vi "All SubFunctions Mod.vi"(4 "מק\"ט המכלל":string, 5 "מספר סידורי":string, 7 "מפעיל":string="ANS", 8 "error":errorcluster, 10 "שם הממסר":string="0410-24534 15A ממסר", 11 "Path for Log":path) -> (0 "error IO":errorcluster)   [LabVIEW 2015]
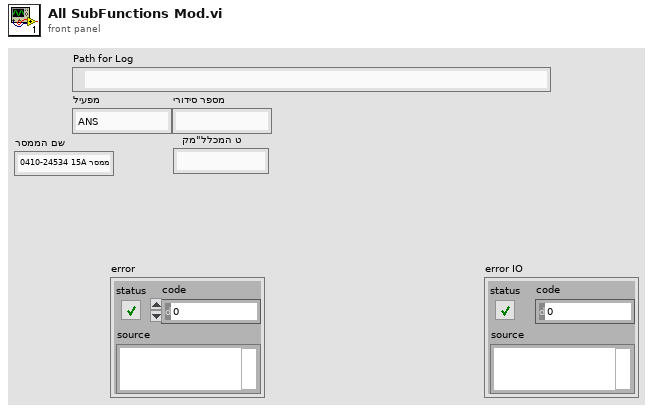
[diagram p1: front panel]
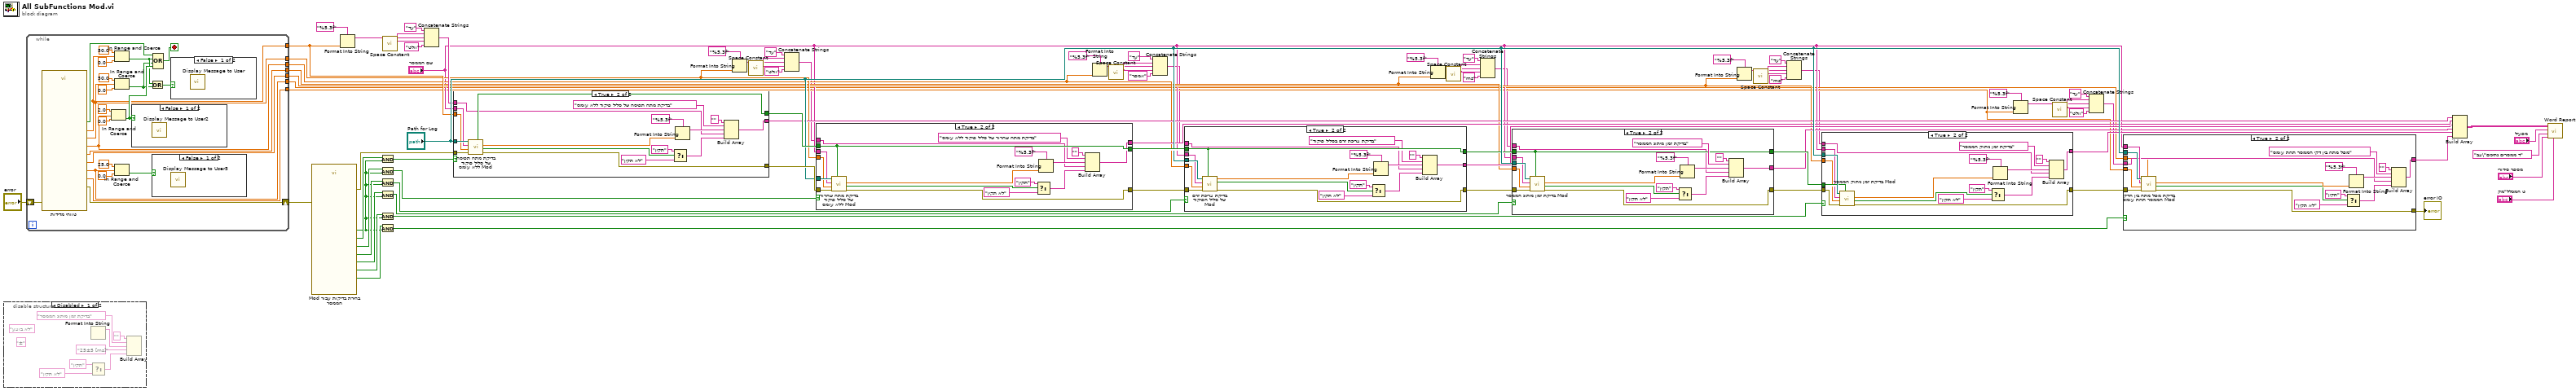
[diagram p0: block diagram]
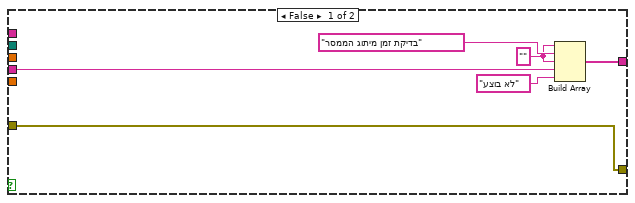
[diagram p6: hidden frame]
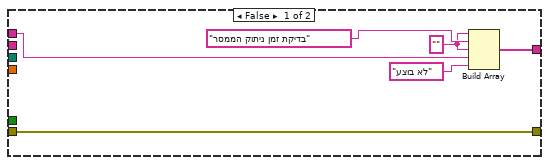
[diagram p7: hidden frame]
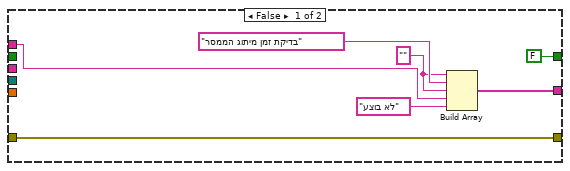
[diagram p8: hidden frame]
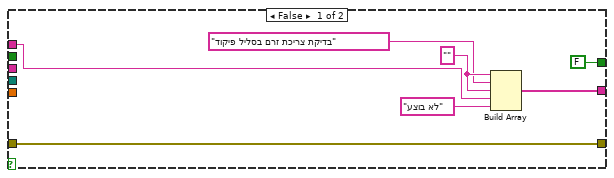
[diagram p9: hidden frame]
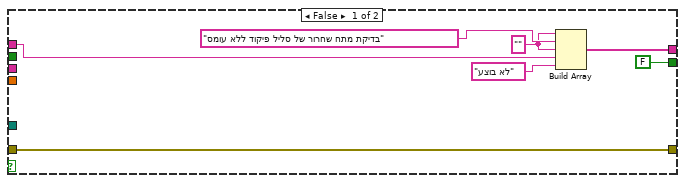
[diagram p10: hidden frame]
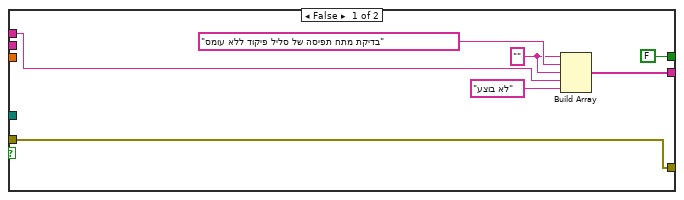
[diagram p11: hidden frame]
diagram:
  n1 = disable-structure shown="Disabled" {
    frame Disabled {
      (unwired) "±"
      (unwired) "לא בוצע"
      n2 = Format Into String() -> (resulting string=w87:string)  [unwired: 4 in, 1 out]
      n3 = Select(t="תקין", f="לא תקין") -> (s? t:f=w89:string)  [unwired: 1 in]
      n4 = Build Array("" ("element"), "בדיקת זמן מיתוג הממסר" ("element"), w87, "25±5 [ms]" ("element"), w89) -> ()  [unwired: 1 out]
    }
    frame Enabled {
    }
  }
  n5 = while {
    shift-right: [w94] -> w45
    shift-left: "error" -> [w95]
    tunnel: [w102] -> w42
    tunnel: [w101] -> w41
    tunnel: [w100] -> w40
    tunnel: [w99] -> w39
    tunnel: [w98] -> w38
    tunnel: [w97] -> w36
    tunnel: [w90] -> w35
    stop <- w106 stop-if-true
    n6 = call "טווחי מדידות"("error in (no error)"=w95) -> ("מפל מתח מקסימלי (V)"=w97:dbl, "זרם הדרוש לבדיקת מפל מתח (A)"=w90:dbl, "זמן ניתוק מקסימלי (mS)"=w98:dbl, "זמן מיתוג מקסימלי (mS)"=w99:dbl, "צריכת זרם מקסימלי (mA)"=w100:dbl, "מתח שחרור מינימלי (V)"=w101:dbl, "מתח תפיסה מקסימלי (V)"=w102:dbl, "OK"=w96:bool, "error out"=w94:errorcluster)  [unwired: 10 in]
    n7 = In Range and Coerce(upper limit=2.0, x=w100, lower limit=0.0) -> (In Range?=w107:bool)  [unwired: 1 out]
    n8 = In Range and Coerce(upper limit=50.0, x=w102, lower limit=0.0) -> (In Range?=w104:bool)  [unwired: 1 out]
    n9 = In Range and Coerce(upper limit=50.0, x=w101, lower limit=0.0) -> (In Range?=w103:bool)  [unwired: 1 out]
    n10 = In Range and Coerce(upper limit=25.0, x=w90, lower limit=0.0) -> (In Range?=w91:bool)  [unwired: 1 out]
    n11 = case shown="False" w107 {
      frame False {
        n12 = call "Display Message to User2"() -> ()  [unwired: 10 in, 2 out]
      }
      frame True {
      }
    }
    n13 = Or(x=w104, y=w103) -> (x .or. y?=w105:bool)
    n14 = case shown="False" w91 {
      frame False {
        n15 = call "Display Message to User3"() -> ()  [unwired: 10 in, 2 out]
      }
      frame True {
      }
    }
    n16 = Compound Arithmetic op=OR(w96, w104, w103, w107) -> (w106:bool)
    n17 = case shown="False" w105 {
      frame False {
        n18 = call "Display Message to User"() -> ()  [unwired: 10 in, 2 out]
      }
      frame True {
      }
    }
  }
  n19 = call "Mod בחירת בדיקות עבור הממסר.vi"("error in (no error)"=w45) -> ("בדיקת מפל מתח בין דקי הממסר תחת עומס"=w66:bool, "בדיקת זמן ניתוק הממסר"=w68:bool, "בדיקת זמן מיתוג הממסר"=w70:bool, "בדיקת צריכת זרם של סליל הפיקוד"=w72:bool, "בדיקת מתח שחרור של סליל פיקוד ללא עומס"=w74:bool, "בדיקת מתח תפיסה של סליל פיקוד ללא עומס"=w64:bool, "OK"=w63:bool, "error out"=w76:errorcluster)  [unwired: 10 in, 1 out]
  n20 = Format Into String(format string="%5.3f", w42) -> (resulting string=w44:string)  [unwired: 2 in, 1 out]
  n21 = And(x=w64, y=w63) -> (x .and. y?=w75:bool)
  n22 = And(x=w74, y=w63) -> (x .and. y?=w73:bool)
  n23 = And(x=w72, y=w63) -> (x .and. y?=w71:bool)
  n24 = And(x=w70, y=w63) -> (x .and. y?=w69:bool)
  n25 = And(x=w68, y=w63) -> (x .and. y?=w67:bool)
  n26 = And(x=w66, y=w63) -> (x .and. y?=w65:bool)
  n27 = call <vilib>:"Space Constant.vi"() -> ("String"=w26:string)
  n28 = Concatenate Strings("עד" ("string"), w26, w44, w26, "וולט" ("string")) -> (w43:string)
  n29 = case shown="True" w75 {
    tunnel: [w120 w137] -> w78
    tunnel: w76 -> [w120 w136]
    tunnel: "Path for Log" -> [_ w135]
    tunnel: [FALSE ("resultUserPrompt") w134] -> w62
    tunnel: [w117 w125] -> w57
    tunnel: "שם הממסר" -> [_ w123]
    tunnel: w43 -> [w114 w122]
    tunnel: w42 -> [_ w121]
    frame False {
      w116 = "" ("element")
      n30 = Build Array(w116, "בדיקת מתח תפיסה של סליל פיקוד ללא עומס" ("element"), w116, w114, "לא בוצע") -> (w117:string[])
    }
    frame True {
      n31 = call "בדיקת מתח תפיסה של סליל פיקוד ללא עומס Mod.vi"("error"=w136, "מתח מקס"=w121, "שם הממסר"=w123, "Path for Log"=w135) -> ("error out"=w137:errorcluster, "מצב ממסר פתוח/סגור"=w131:bool, "מתח סגירת הממסר"=w130:dbl, "resultUserPrompt"=w134:bool)  [unwired: 3 in, 1 out]
      n32 = Select(t="תקין", s=w131, f="לא תקין") -> (s? t:f=w126:string)
      n33 = Format Into String(format string="%5.3f", w130) -> (resulting string=w127:string)  [unwired: 2 in, 1 out]
      n34 = Build Array("" ("element"), "בדיקת מתח תפיסה של סליל פיקוד ללא עומס" ("element"), w127, w122, w126) -> (w125:string[])
    }
  }
  n35 = Format Into String(format string="%5.3f", w41) -> (resulting string=w22:string)  [unwired: 2 in, 1 out]
  n36 = call <vilib>:"Space Constant.vi"() -> ("String"=w23:string)
  n37 = Concatenate Strings("עד" ("string"), w23, w22, w23, "וולט" ("string")) -> (w21:string)
  n38 = case shown="True" w73 {
    tunnel: w78 -> [w144 w161]
    tunnel: [w144 w160] -> w77
    tunnel: "Path for Log" -> [_ w159]
    tunnel: w62 -> [_ w158]
    tunnel: [FALSE ("resultUserPrompt") w158] -> w61
    tunnel: [w139 w149] -> w55
    tunnel: w21 -> [w138 w147]
    tunnel: "שם הממסר" -> [_ w146]
    tunnel: w41 -> [_ w145]
    frame False {
      w140 = "" ("element")
      n39 = Build Array(w140, "בדיקת מתח שחרור של סליל פיקוד ללא עומס" ("element"), w140, w138, "לא בוצע") -> (w139:string[])
    }
    frame True {
      n40 = call "בדיקת מתח שחרור של סליל פיקוד ללא עומס Mod.vi"("resultUserPrompt"=w158, "error"=w161, "זמן סגירה מינימלי"=w145, "שם הממסר"=w146, "Path for Log"=w159) -> ("error out"=w160:errorcluster, "מצב ממסר פתוח/סגור"=w154:bool, "מתח פתיחת הממסר"=w155:dbl)  [unwired: 3 in, 1 out]
      n41 = Select(t="תקין", s=w154, f="לא תקין") -> (s? t:f=w150:string)
      n42 = Format Into String(format string="%5.3f", w155) -> (resulting string=w151:string)  [unwired: 2 in, 1 out]
      n43 = Build Array("" ("element"), "בדיקת מתח שחרור של סליל פיקוד ללא עומס" ("element"), w151, w147, w150) -> (w149:string[])
    }
  }
  n44 = Format Into String(format string="%5.3f", w40) -> (resulting string=w12:string)  [unwired: 2 in, 1 out]
  n45 = call <vilib>:"Space Constant.vi"() -> ("String"=w14:string)
  n46 = Concatenate Strings("עד" ("string"), w14, w12, w14, "אמפר" ("string")) -> (w11:string)
  n47 = case shown="True" w71 {
    tunnel: [w168 w185] -> w81
    tunnel: w77 -> [w168 w184]
    tunnel: "Path for Log" -> [_ w183]
    tunnel: w61 -> [_ w182]
    tunnel: [FALSE ("resultUserPrompt") w182] -> w59
    tunnel: [w163 w173] -> w54
    tunnel: w11 -> [w162 w170]
    tunnel: w40 -> [_ w171]
    tunnel: "שם הממסר" -> [_ w169]
    frame False {
      w166 = "" ("element")
      n48 = Build Array(w166, "בדיקת צריכת זרם בסליל פיקוד" ("element"), w166, w162, "לא בוצע") -> (w163:string[])
    }
    frame True {
      n49 = call "בדיקת צריכת זרם של סליל הפיקוד Mod.vi"("resultUserPrompt"=w182, "error"=w184, "זרם מקסימלי"=w171, "שם הממסר"=w169, "Path for Log"=w183) -> ("error out"=w185:errorcluster, "צריכת זרם בסליל בטווח כן/לא"=w176:bool, "צריכת זרם בסליל"=w177:dbl)  [unwired: 4 in]
      n50 = Select(t="תקין", s=w176, f="לא תקין") -> (s? t:f=w175:string)
      n51 = Format Into String(format string="%5.3f", w177) -> (resulting string=w174:string)  [unwired: 2 in, 1 out]
      n52 = Build Array("" ("element"), "בדיקת צריכת זרם בסליל פיקוד" ("element"), w174, w170, w175) -> (w173:string[])
    }
  }
  n53 = Format Into String(format string="%5.3f", w39) -> (resulting string=w7:string)  [unwired: 2 in, 1 out]
  n54 = call <vilib>:"Space Constant.vi"() -> ("String"=w9:string)
  n55 = Concatenate Strings("עד" ("string"), w9, w7, w9, "ms" ("string")) -> (w6:string)
  n56 = case shown="True" w69 {
    tunnel: w81 -> [w192 w209]
    tunnel: [w192 w208] -> w80
    tunnel: "Path for Log" -> [_ w207]
    tunnel: w59 -> [_ w196]
    tunnel: [FALSE ("resultUserPrompt") w196] -> w58
    tunnel: [w187 w198] -> w53
    tunnel: "שם הממסר" -> [_ w195]
    tunnel: w39 -> [_ w194]
    tunnel: w6 -> [w186 w193]
    frame False {
      w189 = "" ("element")
      n57 = Build Array(w189, "בדיקת זמן מיתוג הממסר" ("element"), w189, w186, "לא בוצע") -> (w187:string[])
    }
    frame True {
      n58 = call "בדיקת זמן מיתוג הממסר Mod.vi"("resultUserPrompt"=w196, "error"=w209, "זמן מיתוג מקסימלי"=w194, "שם הממסר"=w195, "Path for Log"=w207) -> ("error out"=w208:errorcluster, "בטוח כן/לא"=w200:bool, "בדיקת זמן מיתוג הממסר"=w199:dbl)  [unwired: 4 in]
      n59 = Select(t="תקין", s=w200, f="לא תקין") -> (s? t:f=w201:string)
      n60 = Format Into String(format string="%5.3f", w199) -> (resulting string=w202:string)  [unwired: 2 in, 1 out]
      n61 = Build Array("" ("element"), "בדיקת זמן מיתוג הממסר" ("element"), w202, w193, w201) -> (w198:string[])
    }
  }
  n62 = Format Into String(format string="%5.3f", w38) -> (resulting string=w2:string)  [unwired: 2 in, 1 out]
  n63 = call <vilib>:"Space Constant.vi"() -> ("String"=w4:string)
  n64 = Concatenate Strings("עד" ("string"), w4, w2, w4, "ms" ("string")) -> (w1:string)
  n65 = case shown="True" w67 {
    tunnel: w80 -> [w215 w232]
    tunnel: [w215 w231] -> w79
    tunnel: "Path for Log" -> [_ w230]
    tunnel: w58 -> [_ w229]
    tunnel: [w211 w220] -> w52
    tunnel: "שם הממסר" -> [_ w218]
    tunnel: w38 -> [_ w217]
    tunnel: w1 -> [w210 w216]
    frame False {
      w212 = "" ("element")
      n66 = Build Array(w212, "בדיקת זמן ניתוק הממסר" ("element"), w212, w210, "לא בוצע") -> (w211:string[])
    }
    frame True {
      n67 = call "בדיקת זמן ניתוק הממסר Mod.vi"("resultUserPrompt"=w229, "error"=w232, "זמן ניתוק מקסימלי"=w217, "שם הממסר"=w218, "Path for Log"=w230) -> ("error out"=w231:errorcluster, "בטוח כן/לא"=w221:bool, "בדיקת זמן ניתוק הממסר"=w222:dbl)  [unwired: 4 in]
      n68 = Select(t="תקין", s=w221, f="לא תקין") -> (s? t:f=w223:string)
      n69 = Format Into String(format string="%5.3f", w222) -> (resulting string=w224:string)  [unwired: 2 in, 1 out]
      n70 = Build Array("" ("element"), "בדיקת זמן ניתוק הממסר" ("element"), w224, w216, w223) -> (w220:string[])
    }
  }
  n71 = Format Into String(format string="%5.3f", w36) -> (resulting string=w17:string)  [unwired: 2 in, 1 out]
  n72 = call <vilib>:"Space Constant.vi"() -> ("String"=w18:string)
  n73 = Concatenate Strings("עד" ("string"), w18, w17, w18, "וולט" ("string")) -> (w16:string)
  n74 = case shown="True" w65 {
    tunnel: [w238 w255] -> w82
    tunnel: w79 -> [w238 w254]
    tunnel: "Path for Log" -> [_ w253]
    tunnel: [w234 w244] -> w51
    tunnel: "שם הממסר" -> [_ w242]
    tunnel: w36 -> [_ w241]
    tunnel: w16 -> [w233 w240]
    tunnel: w35 -> [_ w239]
    frame False {
      w235 = "" ("element")
      n75 = Build Array(w235, "בדיקת זמן מיתוג הממסר" ("element"), w235, w233, "לא בוצע") -> (w234:string[])
    }
    frame True {
      n76 = call "בדיקת מפל מתח בין הדקי הממסר תחת עומס Mod.vi"("זרם הדרוש"=w239, "error"=w254, "מפל מתח מקסימלי"=w241, "שם הממסר"=w242, "Path for Log"=w253) -> ("error IO"=w255:errorcluster, "In Range?"=w245:bool, "מפל מתח בין דקי הממסר תחת עומס"=w246:dbl)  [unwired: 3 in, 1 out]
      n77 = Select(t="תקין", s=w245, f="לא תקין") -> (s? t:f=w247:string)
      n78 = Format Into String(format string="%5.3f", w246) -> (resulting string=w248:string)  [unwired: 2 in, 1 out]
      n79 = Build Array("" ("element"), "מפל מתח בין דקי הממסר תחת עומס" ("element"), w248, w240, w247) -> (w244:string[])
    }
  }
  "error IO" <- w82
  n80 = Build Array(w57, w55, w54, w53, w52, w51) -> (w56:string[][])
  n81 = call "Word Report.vi"("מק\"ט המכלל"="מק\"ט המכלל", "מספר סידורי"="מספר סידורי", "שם הצב\"ד"="צב\"ד ממסרים נתיכים", "מפעיל"="מפעיל", "Array"=w56) -> ()  [unwired: 7 in]
